vi "MotionProfileRead.vi"() -> ()   [LabVIEW 2018]
uses:
  <vilib>/Utility/file.llb/Read Delimited Spreadsheet (string).vi
panel:
  out "Array":cluster{"X":dbl, "Y":dbl, "Speed":string}[](array[cluster])
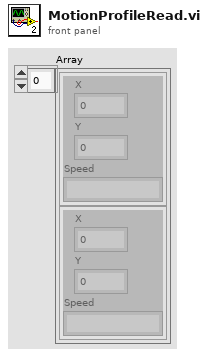
[diagram p1: front panel]
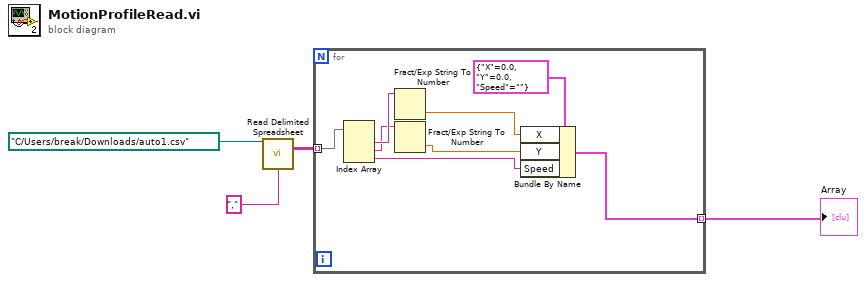
[diagram p0: block diagram]
diagram:
  n1 = call-poly <vilib>:"Read Delimited Spreadsheet.vi"("file path (dialog if empty)"=path "C:/Users/break/Downloads/auto1.csv", "delimiter (\\t)"="," ("delimiter (\\t)")) -> ("all rows"=w3:string[][])  [unwired: 8 in, 5 out]
  n2 = for {
    tunnel: w3 -> [w12] mode=indexing
    tunnel: [w10] -> w1 mode=indexing
    n3 = Index Array(array=w12) -> (element #1=w6:string, element #2=w5:string, element #3=w7:string)  [unwired: 3 in]
    n4 = Fract/Exp String To Number(string=w6) -> (number=w9:dbl)  [unwired: 3 in, 1 out]
    n5 = Fract/Exp String To Number(string=w5) -> (number=w8:dbl)  [unwired: 3 in, 1 out]
    n6 = Bundle By Name(cluster=cluster{"X":dbl, "Y":dbl, "Speed":string} {"X"=0.0, "Y"=0.0, "Speed"=""} ("input cluster"), "X"=w9, "Y"=w8, "Speed"=w7) -> (w10:cluster{"X":dbl, "Y":dbl, "Speed":string})
  }
  "Array" <- w1
